vi "Timer FGV.vi"(7 "Action":T1, 8 "error in (no error)":errorcluster) -> (0 "error out":errorcluster, 3 "Elapsed Time":dbl)   [LabVIEW 2015]
uses:
  Timer Actions.ctl
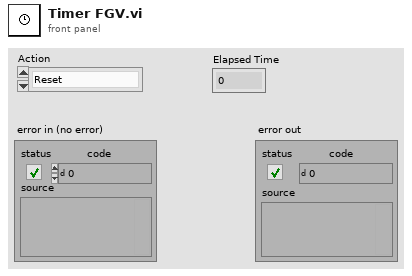
[diagram p1: front panel]
types:
  T1 = typedef "Timer Actions.ctl" = enum16{"Reset", "Get"}
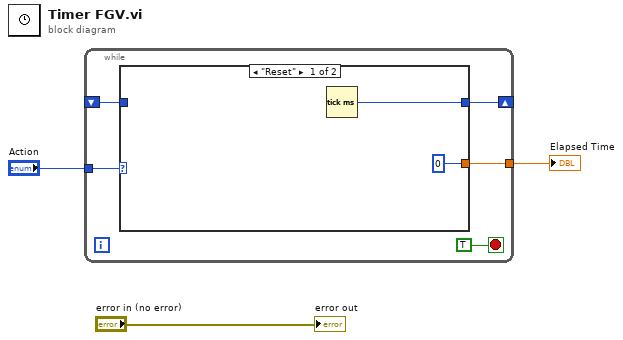
[diagram p0: block diagram]
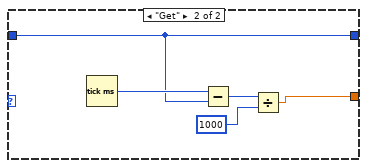
[diagram p2: hidden frame]
diagram:
  n1 = while {
    tunnel: "Action" -> [w7]
    shift-right: [w6] -> _
    shift-left: _ -> [w5]
    tunnel: [w4] -> w3
    stop <- TRUE stop-if-true
    n2 = case shown="\"Reset\"" w7 {
      tunnel: [w10 w14] -> w6
      tunnel: w5 -> [_ w14]
      tunnel: [u32 0 w11] -> w4
      frame "Reset" {
        n3 = Tick Count (ms)() -> (millisecond timer value=w10:u32)
      }
      frame "Get" {
        n4 = Tick Count (ms)() -> (millisecond timer value=w15:u32)
        n5 = Subtract(x=w15, y=w14) -> (x-y=w13:u32)
        n6 = Divide(x=w13, y=u32 1000) -> (x/y=w11:dbl)
      }
    }
  }
  "Elapsed Time" <- w3
  "error out" <- "error in (no error)"
